vi "Accel Filters.vi"(8 "error in (no error)":errorcluster, 11 "Filters":T1[](array[typedef]) {"HP Passband" min=1.0 step=1.0 format="%#.4f"; "LP Stopband" min=1.0 step=1.0 format="%#.4f"; "HP Stopband" min=1.0 step=1.0 format="%#.4f"; "LP Passband" min=1.0 step=1.0 format="%#.4f"}) -> (0 "error out":errorcluster)   [LabVIEW 2018, in "PC UDP Writer.lvlib"]
doc: "This subVI enqueues the named action in to the communications queue along with the input data."
uses:
  PC UDP Writer.lvlib
  Testing UI 3/Private Controls/Cutoff Frequency.ctl
  Private Controls/Module Data.ctl
  Private Controls/Module Action.ctl
  Testing UI 3/Testing UI 3.lvlib
panel:
  # "Highpass Cutoff Frequency"
  # "Lowpass Cutoff Frequency"
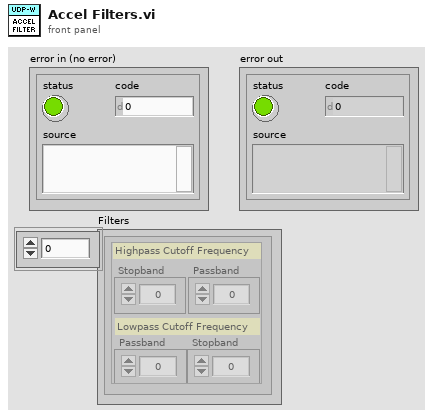
[diagram p1: front panel]
types:
  T1 = typedef "Testing UI 3.lvlib/Cutoff Frequency.ctl" = cluster{"LP Passband":dbl, "HP Stopband":dbl, "LP Stopband":dbl, "HP Passband":dbl}
  T2 = typedef "PC UDP Writer.lvlib/Module Data.ctl" = cluster{"Data":variant, "Action":T3}
  T3 = typedef "PC UDP Writer.lvlib/Module Action.ctl" = enum8{"Init", "Waterfall Select", "Bleed Fuel", "Fuel Pressure Reg", "ECS Demand", "Accel Sensitivities", "Accel Filters", "Shunt Relay", "APU Setup", "APU and ECU Control", "APU Start", "Write", "Error", "Exit"}
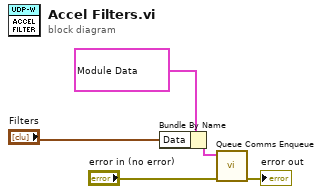
[diagram p0: block diagram]
diagram:
  n1 = Bundle By Name(cluster=T2 {"Data"=variant, "Action"=enum."Accel Filters"} ("element"), "Data"="Filters") -> (w2:T2)
  n2 = call "Queue Comms Enqueue.vi"("error in (no error)"="error in (no error)", "element"=w2) -> ("error out"=→"error out":errorcluster)  [unwired: 9 in]
